vi "WriteLedArray.vi"(8 "error in (no error)":errorcluster, 9 "LED Colors":u32[](array[colorbox]), 10 "Chains":u8[](array[numeric]), 11 "ControlState in":T2 {"ChainMask" format="0x%02x"}) -> (0 "error out":errorcluster, 3 "ControlState out":T2 {"ChainMask" format="0x%02x"}, 5 "Optimization":T1)   [LabVIEW 2020]
uses:
  ControlState.ctl
  ChainState.ctl
  WriteLedArrayStatus.ctl
  Documents/Robotics/swerve-template/Swerve Robot Project Template/LEDs/Implementation/ArduinoSerialBling.lvlib
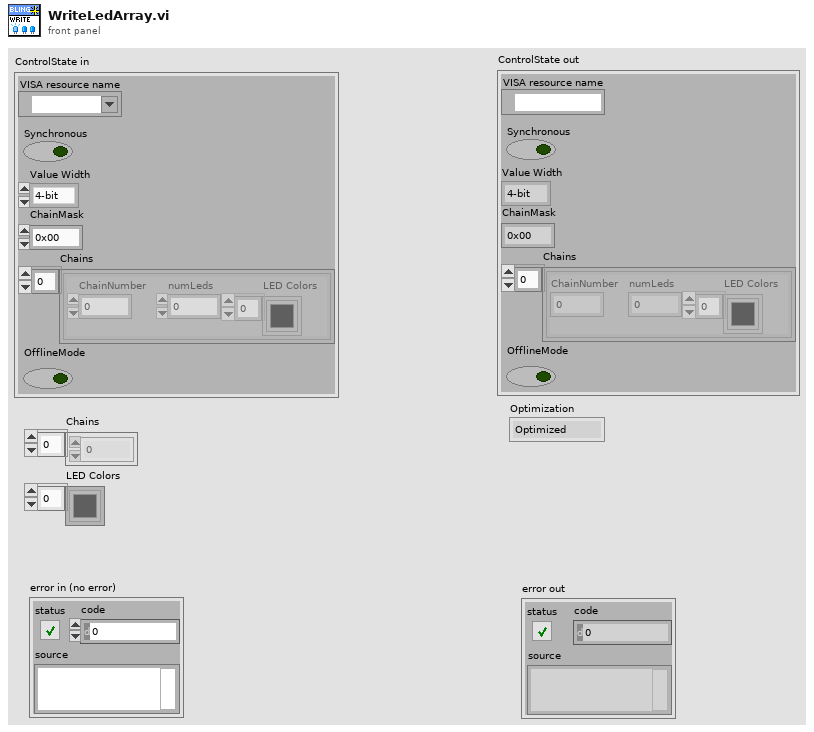
[diagram p1: front panel]
types:
  T1 = typedef "ArduinoSerialBling.lvlib/WriteLedArrayStatus.ctl" = enum16{"Optimized", "Unable to optimize", "No changes", "Error", "Offline"}
  T2 = typedef "ArduinoSerialBling.lvlib/ControlState.ctl" = cluster{"VISA resource name":refnum<visa-resource-name>, "Synchronous":bool, "Value Width":enum16{"4-bit", "8-bit"}, "ChainMask":u8, "Chains":T3[], "OfflineMode":bool}
  T3 = typedef "ArduinoSerialBling.lvlib/ChainState.ctl" = cluster{"ChainNumber":u8, "numLeds":u8, "LED Colors":u32[]}
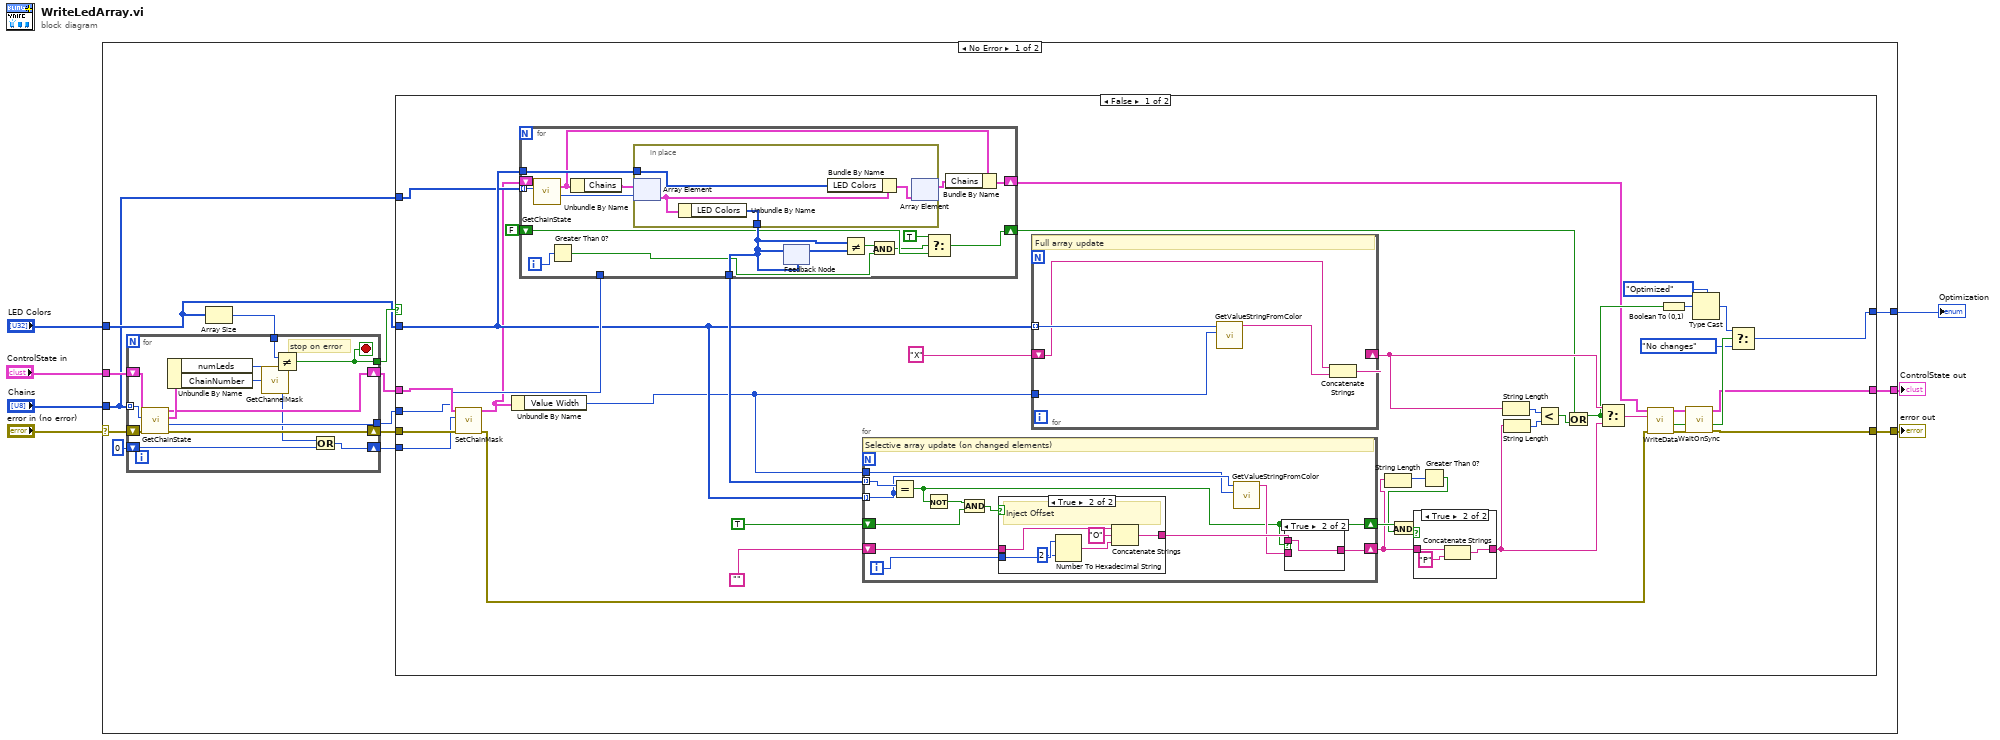
[diagram p0: block diagram]
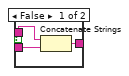
[diagram p3: hidden frame]
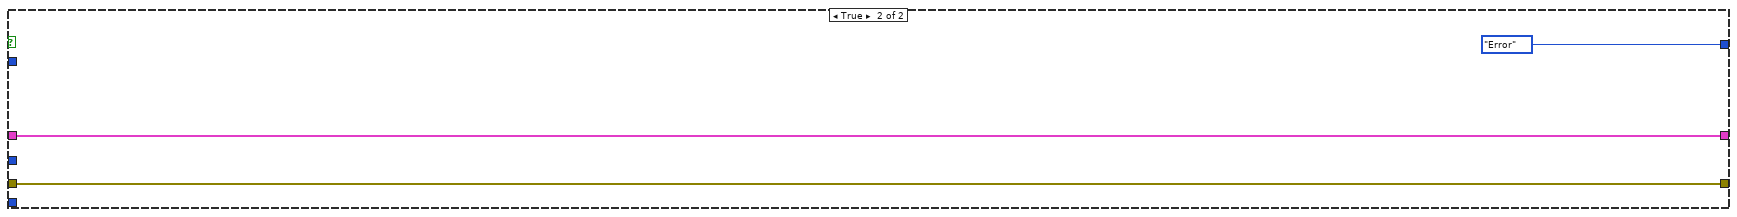
[diagram p5: hidden frame]
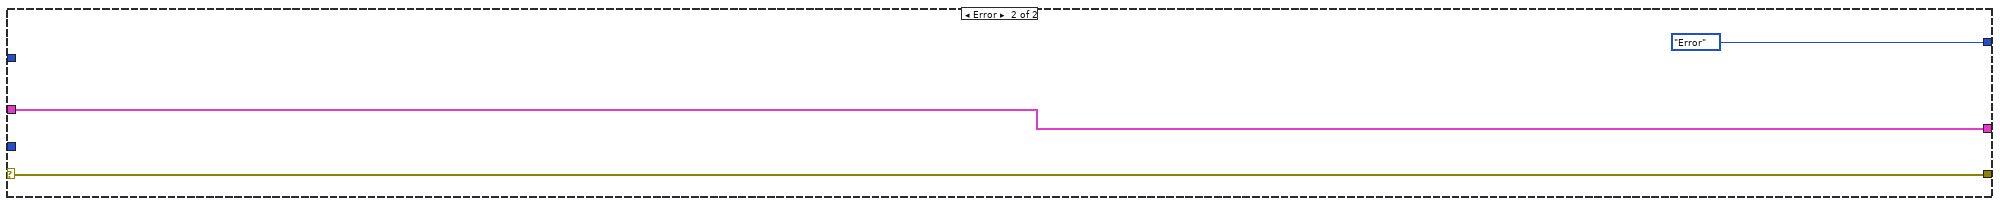
[diagram p6: hidden frame]
diagram:
  n1 = case shown="No Error" "error in (no error)" {
    selector: "error in (no error)" -> [w13 w132]
    tunnel: [w18 w132] -> w7
    tunnel: [w19 w130] -> w6
    tunnel: "LED Colors" -> [w20 _]
    tunnel: [w17 WriteLedArrayStatus."Error" ("Optimization")] -> w4
    tunnel: "ControlState in" -> [w16 w130]
    tunnel: "Chains" -> [w8 _]
    frame No Error {
      n2 = Array Size(array=w20) -> (size(s)=w12:i32)
      n3 = for {
        tunnel: [w26] -> w21
        tunnel: [w34] -> w15
        tunnel: w12 -> [w29]
        shift-right: [w32] -> w14
        shift-left: w16 -> [w35]
        shift-right: [w28] -> w11
        shift-left: w13 -> [w31]
        tunnel: w8 -> [w27] mode=indexing
        shift-right: [w22] -> w9
        shift-left: u8 0 -> [w23]
        stop <- w26 stop-if-true
        # "stop on error"
        n4 = call "GetChainState.vi"("error in (no error)"=w31, "ChainNumber"=w27, "ControlState in"=w35) -> ("error out"=w28:errorcluster, "ChainIndex"=w34:i32, "ChainState"=w33:T3, "ControlState out"=w32:T2)  [unwired: 5 in]
        n5 = Unbundle By Name(w33) -> ("numLeds"=w30:u8, "ChainNumber"=w25:u8)
        n6 = call "GetChannelMask.vi"("ChainNumber"=w25) -> ("ChainMask"=w24:u8)
        n7 = Not Equal?(x=w29, y=w30) -> (x != y?=w26:bool)
        n8 = Or(x=w24, y=w23) -> (x .or. y?=w22:u8)
      }
      n9 = case shown="False" w21 {
        tunnel: w11 -> [w73 w128]
        tunnel: w14 -> [w72 w129]
        tunnel: w20 -> [w60 _]
        tunnel: w15 -> [w71 _]
        tunnel: [w36 w129] -> w19
        tunnel: [w68 w128] -> w18
        tunnel: [w46 WriteLedArrayStatus."Error" ("Optimization")] -> w17
        tunnel: w9 -> [w44 _]
        tunnel: w8 -> [w43 _]
        frame False {
          n10 = call "SetChainMask.vi"("error in (no error)"=w73, "ChainMask"=w44, "ControlState in"=w72) -> ("error out"=w66:errorcluster, "ControlState out"=w42:T2)  [unwired: 7 in]
          n11 = Unbundle By Name(w42) -> ("Value Width"=w57:enum16{"4-bit", "8-bit"})
          n12 = for {
            tunnel: w71 -> [_]
            tunnel: [w84] -> w61
            tunnel: w60 -> [w90]
            tunnel: w43 -> [w89] mode=indexing
            shift-right: [w81] -> w38
            shift-left: FALSE -> [w83]
            shift-right: [w79] -> w37
            shift-left: w42 -> [w88]
            i -> [w77]
            n13 = call "GetChainState.vi"("ChainNumber"=w89, "ControlState in"=w88) -> ("ChainIndex"=w87:i32, "ControlState out"=w80:T2)  [unwired: 6 in, 2 out]
            n14 = Greater Than 0?(x=w77) -> (x > 0?=w75:bool)
            n15 = Unbundle By Name(w80) -> ("Chains"=w86:T3[])
            n16 = in-place {
              in-place-border: w90 -> [w93]
              in-place-border: [w91] -> w84
              n17 = in-place-array #1(w86, w87) -> (w92:T3)
              n18 = Unbundle By Name(w92) -> ("LED Colors"=w91:u32[])
              n19 = Bundle By Name(cluster=w92, "LED Colors"=w93) -> (w94:T3)
              n20 = in-place-array #1(w94) -> (w78:T3[])  [unwired: 1 out]
            }
            n21 = feedback-in #2(w84) -> ()
            n22 = feedback #2(w84) -> (w85:u32[])
            n23 = Not Equal?(x=w84, y=w85) -> (x != y?=w76:bool)
            n24 = And(x=w76, y=w75) -> (x .and. y?=w74:bool)
            n25 = Select(t=TRUE, s=w74, f=w83) -> (s? t:f=w81:bool)
            n26 = Bundle By Name(cluster=w80, "Chains"=w78) -> (w79:T2)
          }
          n27 = for {
            tunnel: w61 -> [w110] mode=indexing
            tunnel: w60 -> [w104] mode=indexing
            shift-right: [w99] -> w52
            shift-left: TRUE -> [w109]
            shift-right: [w100] -> w51
            shift-left: "" -> [w105]
            tunnel: w57 -> [w103]
            i -> [w106]
            # "Selective array update (on changed elements)"
            n28 = Equal?(x=w110, y=w104) -> (x = y?=w99:bool)
            n29 = Not(x=w99) -> (.not. x?=w108:bool)
            n30 = And(x=w108, y=w109) -> (x .and. y?=w107:bool)
            n31 = case shown="True" w107 {
              tunnel: w106 -> [_ w119]
              tunnel: w105 -> [w115 w121]
              tunnel: [w115 w116] -> w102
              frame False {
                # "Continue inserting values"
              }
              frame True {
                # "Inject Offset"
                n32 = Number To Hexadecimal String(1:i16 2 ("width (-)"), 2:w119) -> (0:w117:string)
                n33 = Concatenate Strings(w121, "O" ("string"), w117) -> (w116:string)
              }
            }
            n34 = call "GetValueStringFromColor.vi"("Value Width"=w103, "Color"=w104) -> ("Value String"=w101:string)  [unwired: 9 in]
            n35 = case shown="True" w99 {
              tunnel: w102 -> [w113 w114]
              tunnel: w101 -> [w112 _]
              tunnel: [w111 w114] -> w100
              frame False {
                n36 = Concatenate Strings(w113, w112) -> (w111:string)
              }
              frame True {
              }
            }
          }
          n37 = for {
            tunnel: w60 -> [w126] mode=indexing
            shift-right: [w123] -> w64
            shift-left: "X" -> [w125]
            tunnel: w57 -> [w122]
            # "Full array update"
            n38 = call "GetValueStringFromColor.vi"("Value Width"=w122, "Color"=w126) -> ("Value String"=w124:string)  [unwired: 9 in]
            n39 = Concatenate Strings(w125, w124) -> (w123:string)
          }
          n40 = String Length(string=w51) -> (length=w50:i32)
          n41 = Greater Than 0?(x=w50) -> (x > 0?=w49:bool)
          n42 = And(x=w52, y=w49) -> (x .and. y?=w53:bool)
          n43 = case shown="True" w53 {
            tunnel: w51 -> [w95 w98]
            tunnel: [w95 w96] -> w56
            frame False {
            }
            frame True {
              n44 = Concatenate Strings(w98, "P" ("string")) -> (w96:string)
            }
          }
          n45 = String Length(string=w64) -> (length=w65:i32)
          n46 = String Length(string=w56) -> (length=w63:i32)
          n47 = Less?(x=w65, y=w63) -> (x < y?=w39:bool)
          n48 = Or(x=w38, y=w39) -> (x .or. y?=w40:bool)
          n49 = Select(t=w64, s=w40, f=w56) -> (s? t:f=w62:string)
          n50 = call "WriteData.vi"("error in (no error)"=w66, "Command"=w62, "ControlState in"=w37) -> ("error out"=w70:errorcluster, "Data Written?"=w48:bool, "ControlState out"=w69:T2)  [unwired: 5 in, 1 out]
          n51 = Boolean To (0,1)(Boolean=w40) -> (0, 1=w54:i16)
          n52 = call "WaitOnSync.vi"("error in (no error)"=w70, "Enable"=w48, "ControlState in"=w69) -> ("error out"=w68:errorcluster, "ControlState out"=w36:T2)  [unwired: 7 in]
          n53 = Type Cast(type=WriteLedArrayStatus."Optimized" ("Optimization"), x=w54) -> (*(type *) &x=w47:T1)
          n54 = Select(t=w47, s=w48, f=WriteLedArrayStatus."No changes") -> (s? t:f=w46:T1)
        }
        frame True {
        }
      }
    }
    frame Error {
    }
  }
  "ControlState out" <- w6
  "error out" <- w7
  "Optimization" <- w4
